vi "TimerEngineThread.vi"(11 "DVR":refnum<data-value>) -> ()   [LabVIEW 2017, in "TimerEngine.lvlib" / "TimerEngine.lvclass"]
uses:
  TimerEngine.lvclass
  <vilib>/Platform/TimedLoop/XDataNode/timing_clust.ctl
  <vilib>/Platform/TimedLoop/XDataNode/nitl_modes.ctl
  <vilib>/Platform/TimedLoop/XDataNode/wakeup.ctl
  <vilib>/platform/TimedLoop/XDataNode/XDataNode.xnode
  <vilib>/Platform/TimedLoop/XDataNode/XDNodeRunTimeDep.lvlib
panel:
  out "Period(ms)":i64
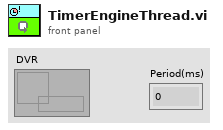
[diagram p1: front panel]
types:
  T1 = typedef "TimerEngine.lvlib/TimerEngine.lvclass/WatchDog--QueueRef.ctl" = refnum<queue>
  T2 = typedef "XDNodeRunTimeDep.lvlib/timing_clust.ctl" = cluster{"Expected End [f-1]":u64, "Actual End [f-1]":u64, "Finished Late? [f-1]":bool, "Expected End [i-1]":u64, "Actual End [i-1]":u64, "Finished Late? [i-1]":bool, "Expected Start [i]":u64, "Actual Start [i]":u64, "Expected Start [f]":u64, "Actual Start [f]":u64, "Source Name":string, "Structure Name":string, "Period":i64, "Deadline":i64, "Offset":i64, "Start":i64, "Priority":i32, "Timeout":i32, "Mode":T3, "Wakeup Reason":T4, "Error":errorcluster, "Source Type":string, "Secondary Source Type":string, "Global End Time":u64, "Global Start Time":u64, "Frame Duration":u64, "Iteration Duration":u64, "Assigned CPU":i32, "I/O Scan Engine Mode":u32}
  T3 = typedef "XDNodeRunTimeDep.lvlib/nitl_modes.ctl" = enum32{"No Change", "Process missed periods, maintain original phase", "Discard missed periods, maintain original phase", "Process missed periods, ignore original phase", "Discard missed periods, ignore original phase"}
  T4 = typedef "XDNodeRunTimeDep.lvlib/wakeup.ctl" = enum32{"Normal", "Aborted", "Asynchronous wakeup", "Timing source error", "Timed loop error", "Timeout"}
  T5 = typedef "TimerEngine.lvlib/TimerEngine.lvclass/Timer-Userevent.ctl" = refnum<user-event>
  T6 = typedef "TimerEngine.lvlib/TimerEngine.lvclass/WatchDogData--Cluster.ctl" = cluster{"TimePeroid(ms)":i32, "ResponeQueue":refnum<queue>, "TimerEngineState":refnum<class>}
  T7 = typedef "TimerEngine.lvlib/TimerEngine.lvclass/Timer-UserEvent.ctl" = refnum<user-event>
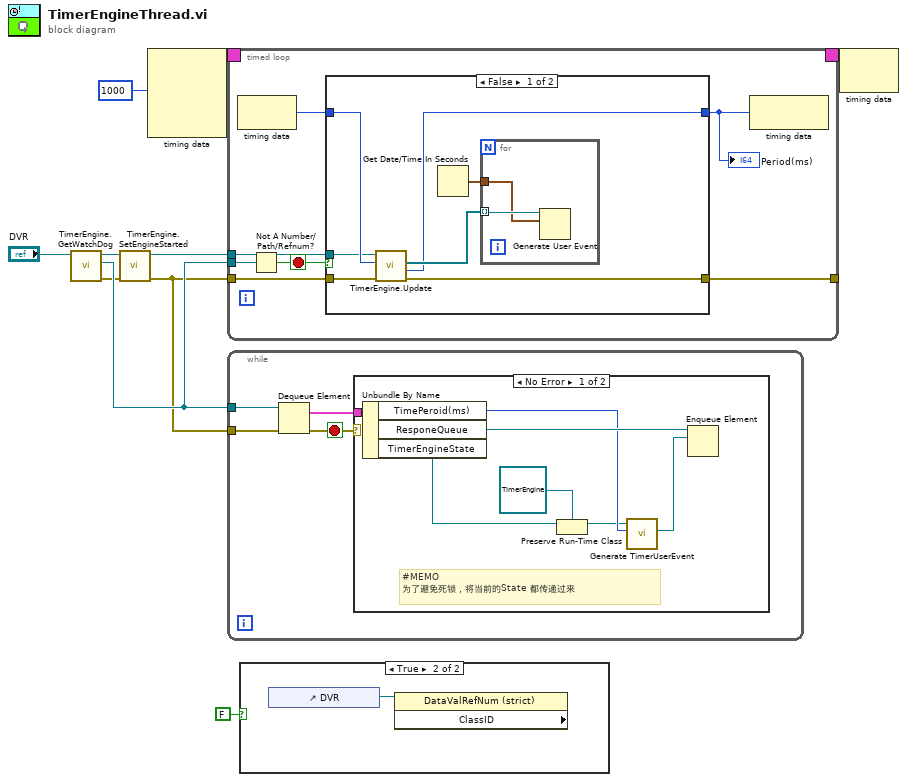
[diagram p0: block diagram]
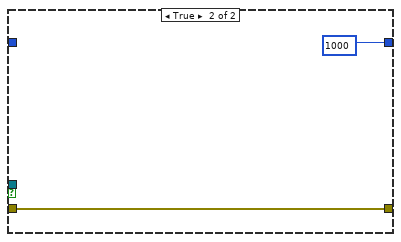
[diagram p4: hidden frame]
diagram:
  n1 = call "TimerEngine.GetWatchDog.vi"("DVR"="DVR") -> ("error out"=w5:errorcluster, "WatchDog"=w6:T1, "DVR 2"=w3:refnum<data-value>)  [unwired: 8 in]
  n2 = call "TimerEngine.SetEngineStarted.vi"("error in (no error)"=w5, "data value reference"=w3) -> ("error out"=w4:errorcluster, "data value reference 2"=w2:refnum<data-value>)  [unwired: 8 in]
  n3 = node-c288(i64 1000 ("Period")) -> (w10:T2)  [unwired: 3 in]
  n4 = timed-loop {
    timing: w10 -> [_]
    timing-out: [_] -> w9
    tunnel: w6 -> [w17]
    tunnel: w4 -> [w16]
    tunnel: [w15] -> _
    tunnel: w2 -> [w13]
    stop <- w12 stop-if-true
    n5 = node-c288() -> (w14:i64)  [unwired: 1 in]
    n6 = Not A Number/Path/Refnum?(number/path/refnum=w17) -> (NaN/Path/Refnum?=w12:bool)
    n7 = case shown="False" w12 {
      tunnel: w16 -> [w24 w27]
      tunnel: [w23 w27] -> w15
      tunnel: w14 -> [w21 _]
      tunnel: [w19 i64 1000 ("Period")] -> w11
      tunnel: w13 -> [w18 _]
      frame False {
        n8 = call "TimerEngine.Update.vi"("error in (no error)"=w24, "TimePassed"=w21, "data value reference"=w18) -> ("error out"=w23:errorcluster, "Cache.TimePeroid(ms)"=w19:i64, "Triggered"=w20:T5[])  [unwired: 5 in, 1 out]
        n9 = Get Date/Time In Seconds() -> (seconds since 1Jan1904=w22:timestamp)
        n10 = for {
          tunnel: w20 -> [w26] mode=indexing
          tunnel: w22 -> [w25]
          n11 = Generate User Event(user event=w26, event data cluster=w25) -> ()  [unwired: 2 in, 2 out]
        }
      }
      frame True {
      }
    }
    "Period(ms)" <- w11
    n12 = node-c288(w11) -> ()  [unwired: 1 out]
  }
  n13 = while {
    tunnel: w6 -> [w37]
    tunnel: w4 -> [w34]
    stop <- w35 stop-if-true
    n14 = Dequeue Element(queue=w37, error in (no error)=w34) -> (element=w36:T6, error out=w35:errorcluster)  [unwired: 1 in, 2 out]
    n15 = case shown="No Error" w35 {
      tunnel: w36 -> [w44 _]
      frame No Error {
        # "#MEMO\n为了避免死锁，将当前的State 都传递过来"
        n16 = Unbundle By Name(w44) -> ("TimePeroid(ms)"=w41:i32, "ResponeQueue"=w43:refnum<queue>, "TimerEngineState"=w42:refnum<class>)
        n17 = Preserve Run-Time Class(object in=w42, 2:refnum<class "TimerEngine.lvclass"> refnum ("TimerEngine.lvlib:TimerEngine.lvclass")) -> (object out=w39:refnum<class "TimerEngine.lvclass">)  [unwired: 1 in, 1 out]
        n18 = call "Generate TimerUserEvent.vi"("TimePeroid(ms)"=w41, "TimerEngine in"=w39) -> ("UserEvent"=w40:T7)  [unwired: 8 in, 1 out]
        n19 = Enqueue Element(queue=w43, element=w40) -> ()  [unwired: 2 in, 3 out]
      }
      frame Error {
      }
    }
  }
  n20 = case shown="True" FALSE {
    frame False {
    }
    frame True {
      n21 = control-ref of="DVR"() -> (w45:refnum<vi>)
      n22 = property class="DataValRefNum (strict)" props=["ClassID"](reference=w45) -> ()  [unwired: 1 in, 3 out]
    }
  }
  n23 = node-c288(w9) -> ()  [unwired: 1 out]
